vi "nanocal -- nuclear schottky goodness V6.vi"(5 "action":T1=enum."onlygrads", 6 "parameters IN":map{T2, dbl}(c390), 7 "weighting strategy":T3, 8 "dz/dω IN (V)":cdb[](array[numeric])=[1.7183506006211996e-05+0.0i, 1.7124360968751133e-05+0.0i, 1.7049104347380084e-05+0.0i, 1.700437896335042e-05+0.0i, 1.6984579723285106e-05+0.0i, 1.702277369054923e-05+0.0i, 1.713094025845651e-05+0.0i, 1.734249707866828e-05+0.0i, 1.768320429215342e-05+0.0i, 1.8195281152538477e-05+0.0i, 1.8917228661806973e-05+0.0i, 1.9897834564883332e-05+0.0i, 2.154104046962704e-05+0.0i, 2.3247799321765792e-05+0.0i, 2.5364678450551808e-05+0.0i, 2.8645788781885885e-05+0.0i, 3.204749554800641e-05+0.0i, 3.783559691555022e-05+0.0i, 4.245015867332296e-05+0.0i, 4.909131821431355e-05+0.0i, 5.511821898441184e-05+0.0i, 6.178843506022867e-05+0.0i, 7.1079604965352e-05+0.0i, 7.922304381453334e-05+0.0i, 8.814778883893872e-05+0.0i, 9.806709148886077e-05+0.0i, 0.00011119043245647465+0.0i, 0.00012253184919712196+0.0i, 0.00013777724317049346+0.0i, 0.0001508081004573332+0.0i, 0.00016547294918783876+0.0i, 0.00018003847596605868+0.0i, 0.00019518361086534857+0.0i, 0.00021134179818259658+0.0i, 0.0002372041782935464+0.0i, 0.00025518143132024254+0.0i, 0.0002835129702467886+0.0i, 0.0003060118087631287+0.0i, 0.00032860772064336976+0.0i, 0.0003492674091322389+0.0i, 0.00037498324855458583+0.0i, 0.00040021078021115026+0.0i, 0.00041969942568205823+0.0i, 0.00044367338947118773+0.0i, 0.0004634793607238068+0.0i, 0.00047921028781215815+0.0i, 0.0004880906353641744+0.0i, 0.0004932212623741357+0.0i, 0.000491476456593048+0.0i, 0.000480893803992059+0.0i, 0.0004535995818650303+0.0i, 0.000417087772881063+0.0i, 0.0003564148692854789+0.0i, 0.0003049201646356487+0.0i, 0.00021260191240459413+0.0i, 0.00011714858948470126+0.0i, 1.675457544365132e-05+0.0i, -6.8674075405897e-05+0.0i, -0.000156473047607305+0.0i, -0.00026709373934749337+0.0i, -0.0003544271565676041+0.0i, -0.00047937600197311275+0.0i, -0.0006086290582260493+0.0i, -0.0007031877411848573+0.0i, -0.0007564526901441745+0.0i, -0.000802489180995596+0.0i, -0.0008414596018105983+0.0i, -0.0008809346482248761+0.0i, -0.0009073902840241921+0.0i, -0.0009264953054508651+0.0i, -0.0009405659412141811+0.0i, -0.000951649722530156+0.0i, -0.0009557485581057351+0.0i, -0.0009558464741053665+0.0i, -0.0009509110176922098+0.0i, -0.0009411315169847015+0.0i, -0.0009303400913929496+0.0i, -0.0009171113529290538+0.0i, -0.0009022111527275027+0.0i, -0.0008813746494947608+0.0i, -0.0008581837971946129+0.0i, -0.0008372063466683705+0.0i, -0.0008165626610594428+0.0i, -0.0007901155435838691+0.0i, -0.0007682834352800848+0.0i, -0.000746231015527196+0.0i, -0.0007238798463130141+0.0i, -0.0007015567569177018+0.0i, -0.000679301954671598+0.0i, -0.0006572001413831251+0.0i, -0.000629855254567978+0.0i, -0.0006083942229188815+0.0i, -0.0005768631156754208+0.0i, -0.0005562177438951648+0.0i, -0.0005359092039599222+0.0i, -0.0005145186443378148+0.0i, -0.0004951602053444319+0.0i, -0.00047624970229075174+0.0i, -0.0004577401041527736+0.0i, -0.00043519037796120065+0.0i], 9 "Voltage IN (V)":cdb[](array[numeric])=[1.7183506006211996e-05+0.0i, 1.7124360968751133e-05+0.0i, 1.7049104347380084e-05+0.0i, 1.700437896335042e-05+0.0i, 1.6984579723285106e-05+0.0i, 1.702277369054923e-05+0.0i, 1.713094025845651e-05+0.0i, 1.734249707866828e-05+0.0i, 1.768320429215342e-05+0.0i, 1.8195281152538477e-05+0.0i, 1.8917228661806973e-05+0.0i, 1.9897834564883332e-05+0.0i, 2.154104046962704e-05+0.0i, 2.3247799321765792e-05+0.0i, 2.5364678450551808e-05+0.0i, 2.8645788781885885e-05+0.0i, 3.204749554800641e-05+0.0i, 3.783559691555022e-05+0.0i, 4.245015867332296e-05+0.0i, 4.909131821431355e-05+0.0i, 5.511821898441184e-05+0.0i, 6.178843506022867e-05+0.0i, 7.1079604965352e-05+0.0i, 7.922304381453334e-05+0.0i, 8.814778883893872e-05+0.0i, 9.806709148886077e-05+0.0i, 0.00011119043245647465+0.0i, 0.00012253184919712196+0.0i, 0.00013777724317049346+0.0i, 0.0001508081004573332+0.0i, 0.00016547294918783876+0.0i, 0.00018003847596605868+0.0i, 0.00019518361086534857+0.0i, 0.00021134179818259658+0.0i, 0.0002372041782935464+0.0i, 0.00025518143132024254+0.0i, 0.0002835129702467886+0.0i, 0.0003060118087631287+0.0i, 0.00032860772064336976+0.0i, 0.0003492674091322389+0.0i, 0.00037498324855458583+0.0i, 0.00040021078021115026+0.0i, 0.00041969942568205823+0.0i, 0.00044367338947118773+0.0i, 0.0004634793607238068+0.0i, 0.00047921028781215815+0.0i, 0.0004880906353641744+0.0i, 0.0004932212623741357+0.0i, 0.000491476456593048+0.0i, 0.000480893803992059+0.0i, 0.0004535995818650303+0.0i, 0.000417087772881063+0.0i, 0.0003564148692854789+0.0i, 0.0003049201646356487+0.0i, 0.00021260191240459413+0.0i, 0.00011714858948470126+0.0i, 1.675457544365132e-05+0.0i, -6.8674075405897e-05+0.0i, -0.000156473047607305+0.0i, -0.00026709373934749337+0.0i, -0.0003544271565676041+0.0i, -0.00047937600197311275+0.0i, -0.0006086290582260493+0.0i, -0.0007031877411848573+0.0i, -0.0007564526901441745+0.0i, -0.000802489180995596+0.0i, -0.0008414596018105983+0.0i, -0.0008809346482248761+0.0i, -0.0009073902840241921+0.0i, -0.0009264953054508651+0.0i, -0.0009405659412141811+0.0i, -0.000951649722530156+0.0i, -0.0009557485581057351+0.0i, -0.0009558464741053665+0.0i, -0.0009509110176922098+0.0i, -0.0009411315169847015+0.0i, -0.0009303400913929496+0.0i, -0.0009171113529290538+0.0i, -0.0009022111527275027+0.0i, -0.0008813746494947608+0.0i, -0.0008581837971946129+0.0i, -0.0008372063466683705+0.0i, -0.0008165626610594428+0.0i, -0.0007901155435838691+0.0i, -0.0007682834352800848+0.0i, -0.000746231015527196+0.0i, -0.0007238798463130141+0.0i, -0.0007015567569177018+0.0i, -0.000679301954671598+0.0i, -0.0006572001413831251+0.0i, -0.000629855254567978+0.0i, -0.0006083942229188815+0.0i, -0.0005768631156754208+0.0i, -0.0005562177438951648+0.0i, -0.0005359092039599222+0.0i, -0.0005145186443378148+0.0i, -0.0004951602053444319+0.0i, -0.00047624970229075174+0.0i, -0.0004577401041527736+0.0i, -0.00043519037796120065+0.0i], 10 "ω (rad/sec)":dbl[](array[numeric])=[32012.991918577427, 32390.261658505893, 32466.39798177853, 32499.14340521798, 32517.39286113775, 32529.046092051318, 32537.14525712326, 32543.111142615544, 32547.696343954158, 32551.33675949651, 32554.302325209504, 32556.769142360055, 32558.856995237307, 32560.650202739795, 32562.209843476354, 32563.58125099723, 32564.7987833122, 32565.88895894197, 32566.872575330308, 32567.766175404246, 32568.583086316496, 32569.334166794306, 32570.02835688638, 32570.673085530187, 32571.274580490695, 32571.838104118455, 32572.36813539066, 32572.868514009202, 32573.342552524307, 32573.793126289274, 32574.222746575288, 32574.633618125405, 32575.027687968828, 32575.40668442971, 32575.772149741057, 32576.12546690325, 32576.467883345118, 32576.800529469096, 32577.124435064776, 32577.440543590797, 32577.749724325146, 32578.052781957467, 32578.35046682089, 32578.643482565894, 32578.932492128843, 32579.218126471686, 32579.500987779396, 32579.781656707495, 32580.06069600583, 32580.338656060805, 32580.616078519142, 32580.89350097748, 32581.171461032456, 32581.45050033079, 32581.73116925889, 32582.0140305666, 32582.29966469628, 32582.58867447239, 32582.88169000423, 32583.179375080817, 32583.48243271314, 32583.791613234323, 32584.10772197351, 32584.43162756919, 32584.764273480003, 32585.106690135035, 32585.460007297228, 32585.825472395412, 32586.204468856296, 32586.59853891288, 32587.009410462997, 32587.439030535847, 32587.889604513977, 32588.363642815923, 32588.86402143446, 32589.39405291983, 32589.957576334426, 32590.559071508098, 32591.203800151903, 32591.897990030815, 32592.64907072179, 32593.46598163404, 32594.359581707977, 32595.343197883154, 32596.433373726086, 32597.650906041054, 32599.022313348767, 32600.58195429849, 32602.375161800977, 32604.46301467823, 32606.929831615616, 32609.895397541775, 32613.535812870963, 32618.12101442274, 32624.086899701866, 32632.186064986967, 32643.839295900536, 32662.088751820305, 32694.834175046595, 32770.97049853239]) -> (0 "R norm":dbl=-1.0, 1 "G":dbl=-1.0, 2 "R(ω) out":cdb[](array[numeric])=[1.7183506006211996e-05+0.0i, 1.7124360968751133e-05+0.0i, 1.7049104347380084e-05+0.0i, 1.700437896335042e-05+0.0i, 1.6984579723285106e-05+0.0i, 1.702277369054923e-05+0.0i, 1.713094025845651e-05+0.0i, 1.734249707866828e-05+0.0i, 1.768320429215342e-05+0.0i, 1.8195281152538477e-05+0.0i, 1.8917228661806973e-05+0.0i, 1.9897834564883332e-05+0.0i, 2.154104046962704e-05+0.0i, 2.3247799321765792e-05+0.0i, 2.5364678450551808e-05+0.0i, 2.8645788781885885e-05+0.0i, 3.204749554800641e-05+0.0i, 3.783559691555022e-05+0.0i, 4.245015867332296e-05+0.0i, 4.909131821431355e-05+0.0i, 5.511821898441184e-05+0.0i, 6.178843506022867e-05+0.0i, 7.1079604965352e-05+0.0i, 7.922304381453334e-05+0.0i, 8.814778883893872e-05+0.0i, 9.806709148886077e-05+0.0i, 0.00011119043245647465+0.0i, 0.00012253184919712196+0.0i, 0.00013777724317049346+0.0i, 0.0001508081004573332+0.0i, 0.00016547294918783876+0.0i, 0.00018003847596605868+0.0i, 0.00019518361086534857+0.0i, 0.00021134179818259658+0.0i, 0.0002372041782935464+0.0i, 0.00025518143132024254+0.0i, 0.0002835129702467886+0.0i, 0.0003060118087631287+0.0i, 0.00032860772064336976+0.0i, 0.0003492674091322389+0.0i, 0.00037498324855458583+0.0i, 0.00040021078021115026+0.0i, 0.00041969942568205823+0.0i, 0.00044367338947118773+0.0i, 0.0004634793607238068+0.0i, 0.00047921028781215815+0.0i, 0.0004880906353641744+0.0i, 0.0004932212623741357+0.0i, 0.000491476456593048+0.0i, 0.000480893803992059+0.0i, 0.0004535995818650303+0.0i, 0.000417087772881063+0.0i, 0.0003564148692854789+0.0i, 0.0003049201646356487+0.0i, 0.00021260191240459413+0.0i, 0.00011714858948470126+0.0i, 1.675457544365132e-05+0.0i, -6.8674075405897e-05+0.0i, -0.000156473047607305+0.0i, -0.00026709373934749337+0.0i, -0.0003544271565676041+0.0i, -0.00047937600197311275+0.0i, -0.0006086290582260493+0.0i, -0.0007031877411848573+0.0i, -0.0007564526901441745+0.0i, -0.000802489180995596+0.0i, -0.0008414596018105983+0.0i, -0.0008809346482248761+0.0i, -0.0009073902840241921+0.0i, -0.0009264953054508651+0.0i, -0.0009405659412141811+0.0i, -0.000951649722530156+0.0i, -0.0009557485581057351+0.0i, -0.0009558464741053665+0.0i, -0.0009509110176922098+0.0i, -0.0009411315169847015+0.0i, -0.0009303400913929496+0.0i, -0.0009171113529290538+0.0i, -0.0009022111527275027+0.0i, -0.0008813746494947608+0.0i, -0.0008581837971946129+0.0i, -0.0008372063466683705+0.0i, -0.0008165626610594428+0.0i, -0.0007901155435838691+0.0i, -0.0007682834352800848+0.0i, -0.000746231015527196+0.0i, -0.0007238798463130141+0.0i, -0.0007015567569177018+0.0i, -0.000679301954671598+0.0i, -0.0006572001413831251+0.0i, -0.000629855254567978+0.0i, -0.0006083942229188815+0.0i, -0.0005768631156754208+0.0i, -0.0005562177438951648+0.0i, -0.0005359092039599222+0.0i, -0.0005145186443378148+0.0i, -0.0004951602053444319+0.0i, -0.00047624970229075174+0.0i, -0.0004577401041527736+0.0i, -0.00043519037796120065+0.0i], 3 "dG / d log α   OUT":map{T2, dbl}(c390), 4 "d2G / d log α d log  β  map  OUT":map{i32[], dbl}(c390))   [LabVIEW 2021]
uses:
  nanocal-goodness-weighting-strategy.ctl
  3-lorentzian-parameters.ctl
  3-lorentzian-heat-response action.ctl
  <vilib>/Utility/miscctls.llb/LVMapReplaceAction.ctl
  <vilib>/Analysis/_algsub.llb/Matrix Norm Type.ctl
  <vilib>/Analysis/baseanly.llb/Matrix Type of Inverse Matrix.ctl
  <vilib>/Analysis/baseanly.llb/Real A x B.vi
  <vilib>/Analysis/_algsub.llb/Real Matrix Norm.vi
  <vilib>/Analysis/Matrix/Numeric/Conversions/Array To Matrix - RA2.vi
  <vilib>/Analysis/baseanly.llb/Real Inverse Matrix.vi
  <vilib>/Analysis/Matrix/Numeric/Conversions/Array To Matrix - RA.vi
  <vilib>/Analysis/Matrix/Numeric/Conversions/Matrix To Array - RM.vi
  <vilib>/Analysis/Matrix/NI_Matrix.lvlib
  <vilib>/Analysis/NI_AALBase.lvlib
  <vilib>/Analysis/NI_AALPro.lvlib
panel:
  out "d2G / d log α d log  β  matrix OUT":dbl[](array[numeric])
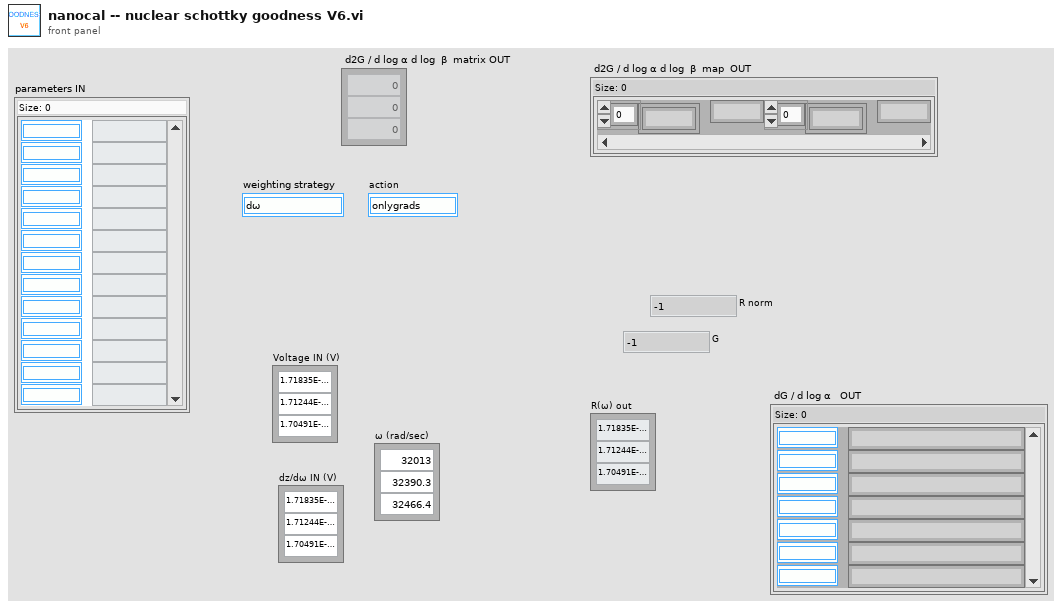
[diagram p1: front panel]
types:
  T1 = typedef "3-lorentzian-heat-response action.ctl" = enum16{"calc R", "create string", "calc m1m2m3", "dζ", "dT1", "dτS", "dτN", "dτC", "d-all", "dκ0", "T(K)", "m1", "m2", "m3", "parse string", "θ (deg)", "B (T)", "onlygrads", "newton", "create emty string", "simple2nd", "calc R2"}
  T2 = typedef "3-lorentzian-parameters.ctl" = enum16{"ζ", "τ1", "τS", "τN", "τC", "κ0", "m1", "m2", "m3", "T (K)", "B (T)", "θ (deg)", "side (S|R)", "set of (B|T)", "Re(offset)", "Im(offset)", "στ1", "στ1-", "στ1+", "στS", "στS-", "στS+", "στN", "στN-", "στN+", "τ11", "τ12", "τ21", "τ22", "τN1", "τN2"}
  T3 = typedef "nanocal-goodness-weighting-strategy.ctl" = enum16{"dω", "dω √(|dz/dω|)", "dω |dz/dω|", "phase", "andreas", "sum", "anti-andr", "ark"}
  T4 = typedef "LVMapReplaceAction.ctl" = enum32{"Modify Entry only if found", "Add or Modify Entry", "Delete Entry"}
  T5 = typedef "NI_AALBase.lvlib/Matrix Type of Inverse Matrix.ctl" = enum32{"General", "Positive Definite", "Lower Triangular", "Upper Triangular"}
  T6 = typedef "NI_AALPro.lvlib/Matrix Norm Type.ctl" = i32
  T7 = typedef "NI_Matrix.lvlib/RealMatrix.ctl" = dbl[][]
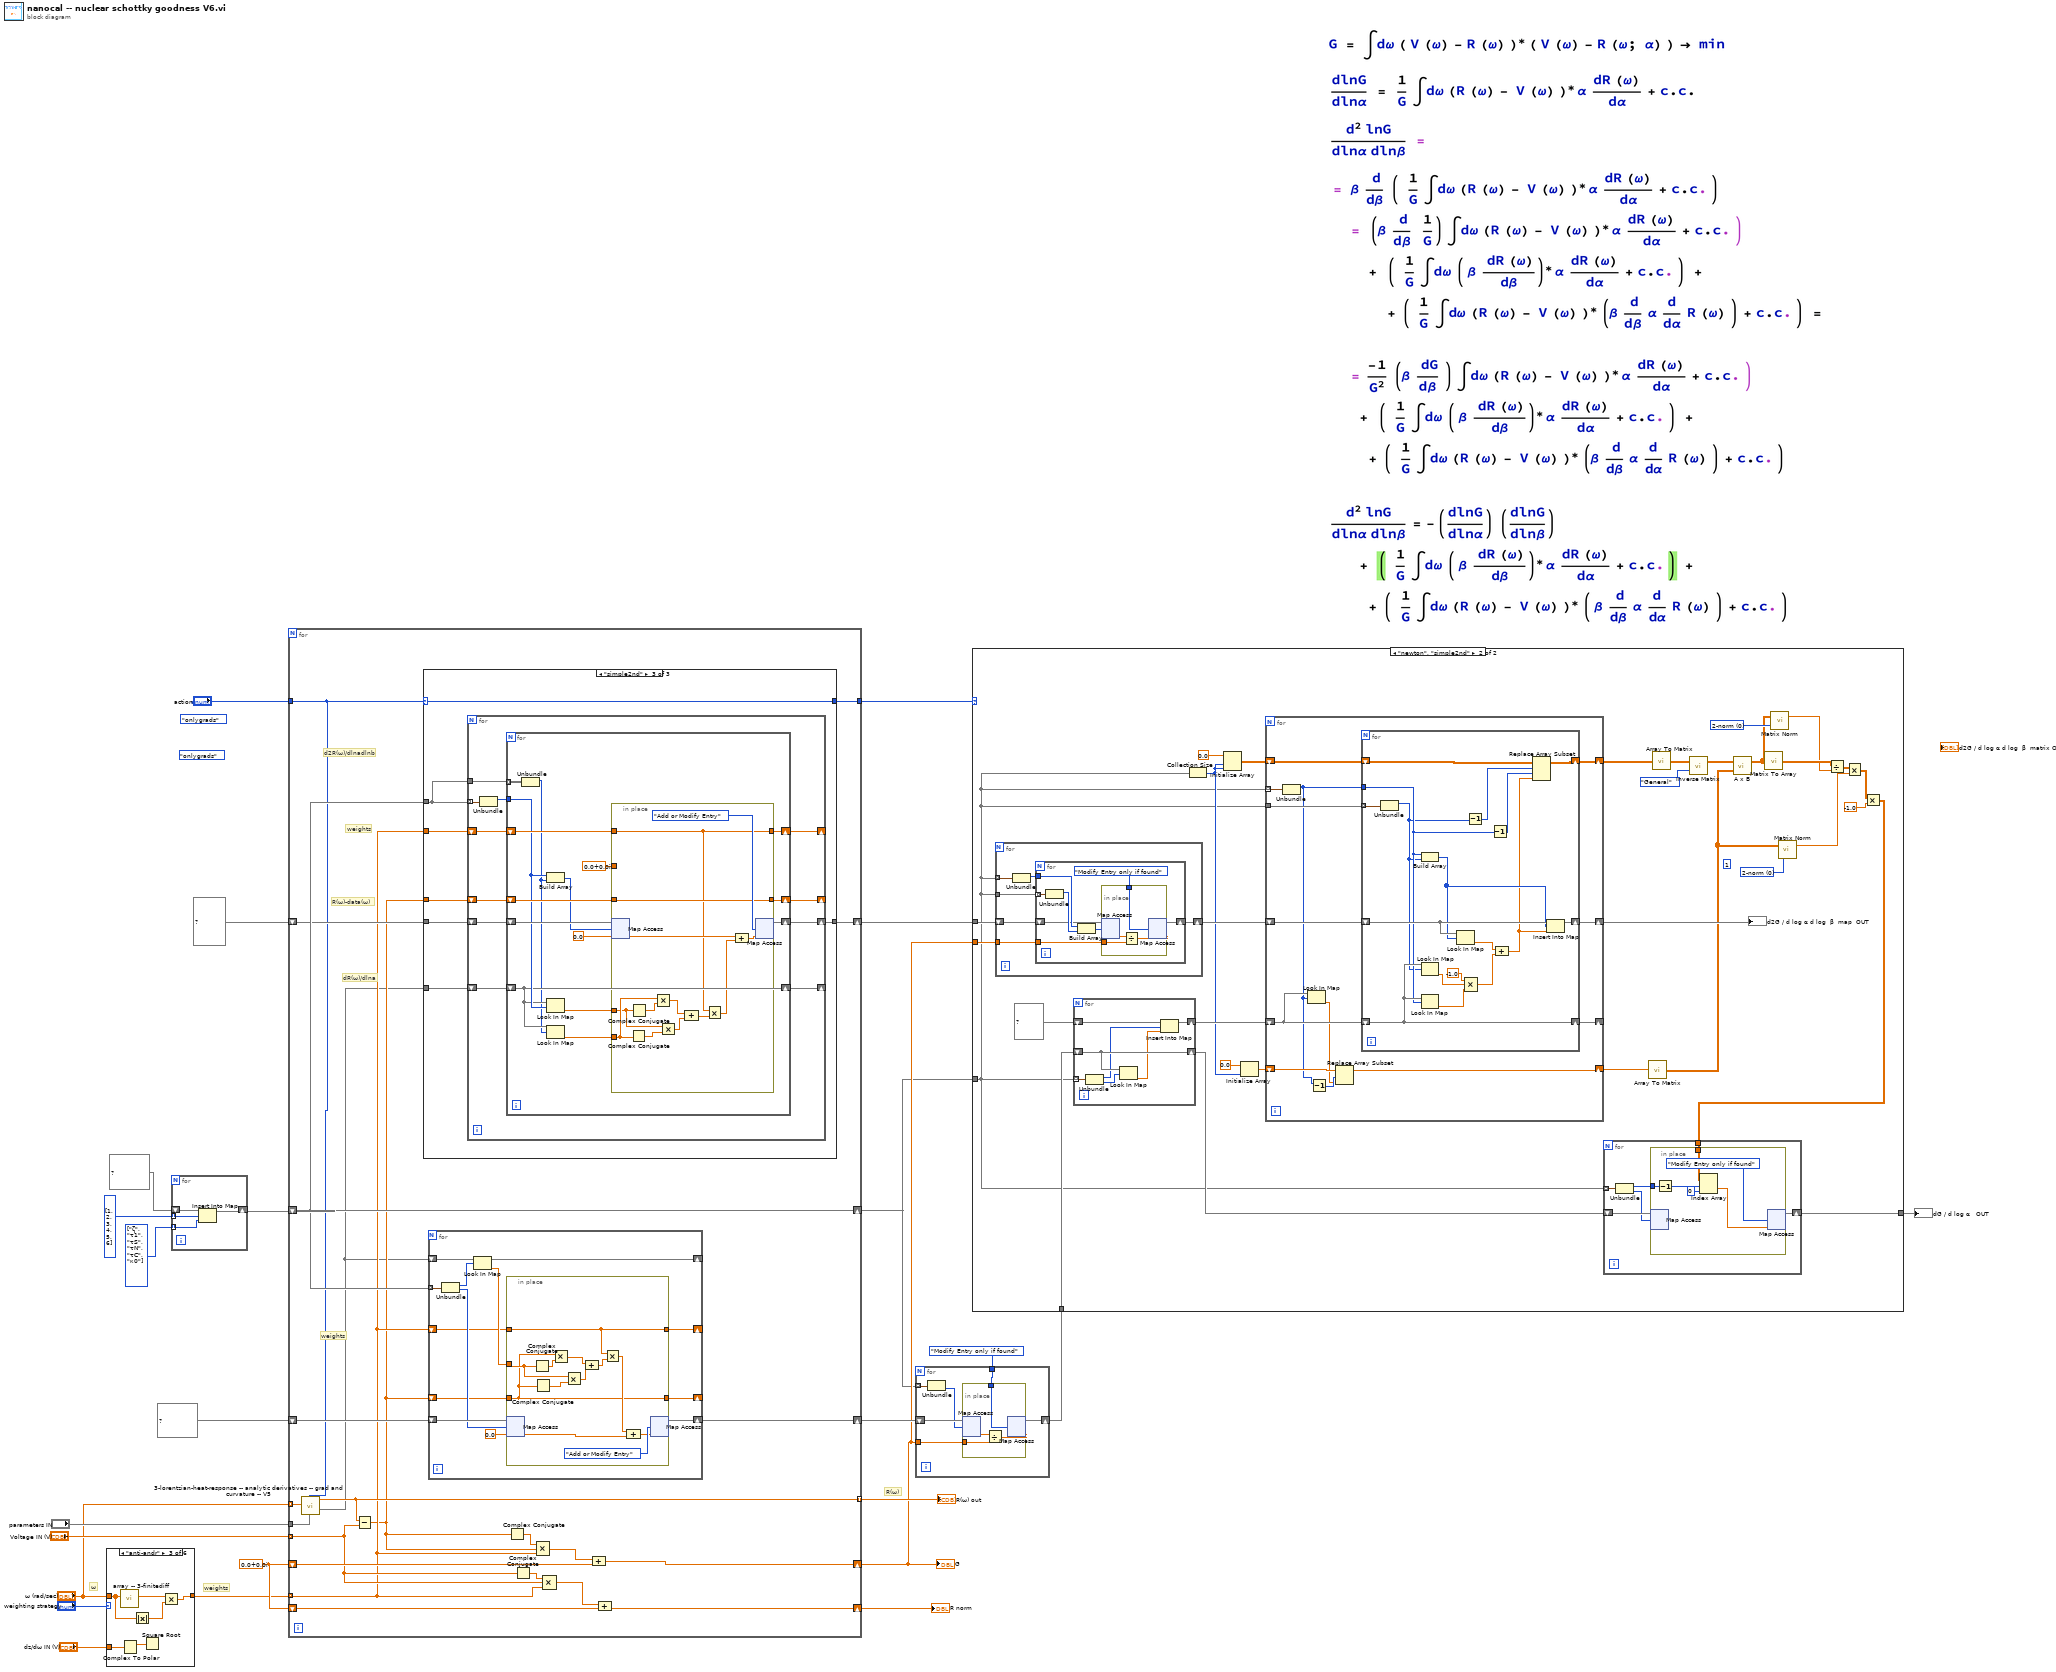
[diagram p0: block diagram]
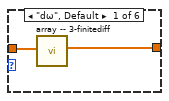
[diagram p3: hidden frame]
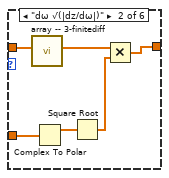
[diagram p4: hidden frame]
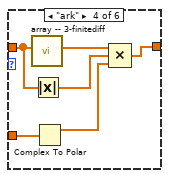
[diagram p5: hidden frame]
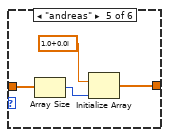
[diagram p6: hidden frame]
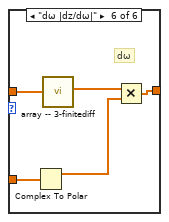
[diagram p7: hidden frame]
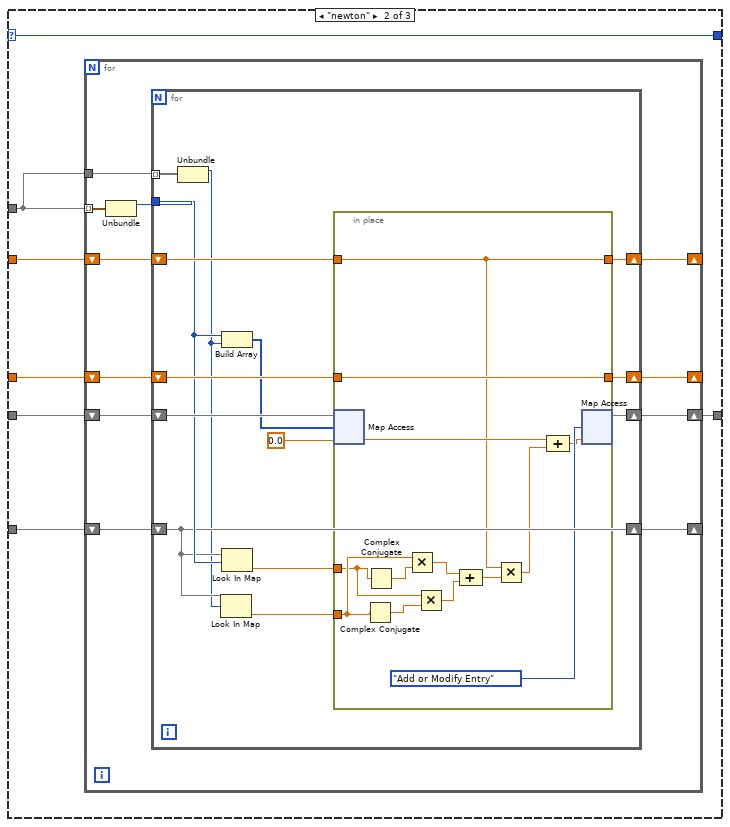
[diagram p9: hidden frame]
diagram:
  (unwired) 3-lorentzian-heat-response_action."onlygrads" ("action")
  (unwired) 3-lorentzian-heat-response_action."onlygrads" ("action")
  w14 = cdb 0.0+0.0i ("y")
  w19 = T2[] [enum."ζ", enum."τ1", enum."τS", enum."τN", enum."τC", enum."κ0"] items=["ζ", "τ1", "τS", "τN", "τC", "κ0", "m1", "m2", "m3", "T (K)", "B (T)", "θ (deg)", "side (S|R)", "set of (B|T)", "Re(offset)", "Im(offset)", "στ1", "στ1-", "στ1+", "στS", "στS-", "στS+", "στN", "στN-", "στN+", "τ11", "τ12", "τ21", "τ22", "τN1", "τN2"]
  # "weights"
  # "R(ω)"
  # "ω"
  n1 = case shown="\"anti-andr\"" "weighting strategy" {
    tunnel: "dz/dω IN (V)" -> [_ w32 w38 w44 _ w53]
    tunnel: "ω (rad/sec)" -> [w26 w28 w34 w41 w48 w52]
    tunnel: [w25 w27 w35 w42 w45 w49] -> w3
    frame "dω", Default {
      n2 = call "array -- 3-finitediff.vi"("ω (rad/sec)"=w26) -> ("dω (rad/sec)"=w25:cdb[])  [unwired: 10 in]
    }
    frame "dω √(|dz/dω|)" {
      n3 = call "array -- 3-finitediff.vi"("ω (rad/sec)"=w28) -> ("dω (rad/sec)"=w30:cdb[])  [unwired: 10 in]
      n4 = Complex To Polar(r * e^(i*theta)=w32) -> (r=w31:dbl[])  [unwired: 1 out]
      n5 = Square Root(x=w31) -> (sqrt(x)=w29:dbl[])
      n6 = Multiply(x=w30, y=w29) -> (x*y=w27:cdb[])
    }
    frame "anti-andr" {
      n7 = call "array -- 3-finitediff.vi"("ω (rad/sec)"=w34) -> ("dω (rad/sec)"=w36:cdb[])  [unwired: 10 in]
      n8 = Complex To Polar(r * e^(i*theta)=w38) -> (r=w37:dbl[])  [unwired: 1 out]
      n9 = Absolute Value(x=w34) -> (abs(x)=w33:dbl[])
      n10 = Square Root(x=w37) -> ()  [unwired: 1 out]
      n11 = Multiply(x=w36, y=w33) -> (x*y=w35:cdb[])
    }
    frame "ark" {
      n12 = call "array -- 3-finitediff.vi"("ω (rad/sec)"=w41) -> ("dω (rad/sec)"=w43:cdb[])  [unwired: 10 in]
      n13 = Absolute Value(x=w41) -> (abs(x)=w40:dbl[])
      n14 = Complex To Polar(r * e^(i*theta)=w44) -> (r=w39:dbl[])  [unwired: 1 out]
      n15 = Compound Arithmetic op=MULTIPLY(w43, w40, w39) -> (w42:cdb[])
    }
    frame "andreas" {
      n16 = Array Size(array=w48) -> (size(s)=w47:i32)
      n17 = Initialize Array(cdb 1.0+0.0i ("y"), w47) -> (w45:cdb[])
    }
    frame "dω |dz/dω|" {
      # "dω"
      n18 = Complex To Polar(r * e^(i*theta)=w53) -> (r=w51:dbl[])  [unwired: 1 out]
      n19 = call "array -- 3-finitediff.vi"("ω (rad/sec)"=w52) -> ("dω (rad/sec)"=w50:cdb[])  [unwired: 10 in]
      n20 = Multiply(x=w50, y=w51) -> (x*y=w49:cdb[])
    }
  }
  n21 = for {
    tunnel: w19 -> [w54] mode=indexing
    shift-right: [w56] -> w12
    shift-left: map{i32, T2} {} ("parameters IN") -> [w57]
    tunnel: i32[] [1, 2, 3, 4, 5, 6] -> [w55] mode=indexing
    n22 = Insert Into Map(map in=w57, key=w55, value=w54) -> (map out=w56:map{i32, T2})  [unwired: 2 out]
  }
  n23 = for {
    tunnel: "ω (rad/sec)" -> [w78] mode=indexing
    tunnel: [w77] -> w21 mode=indexing
    tunnel: "parameters IN" -> [w79]
    tunnel: "Voltage IN (V)" -> [w66] mode=indexing
    tunnel: w3 -> [w62] mode=indexing
    shift-right: [w75] -> w15
    shift-left: map{T2, dbl} {} ("parameters IN") -> [w76]
    shift-right: [w65] -> w7
    shift-left: w12 -> [w65]
    shift-right: [w71] -> w8
    shift-left: w14 -> [w72]
    shift-right: [w67] -> w13
    shift-left: w14 -> [w68]
    shift-right: [w63] -> w9
    shift-left: map{i32[], dbl} {} ("parameters IN") -> [w64]
    tunnel: "action" -> [w59]
    tunnel: [w58] -> w5
    # "R(ω)-data(ω)"
    # "weights"
    # "dR(ω)/dlna"
    # "d2R(ω)/dlnadlnb"
    # "weights"
    n24 = call "3-lorentzian-heat-response -- analytic derivatives -- grad and curvature -- V5.vi"("parameters map  IN"=w79, "action"=w59, "ω (rad/sec)"=w78) -> ("grad map  out"=w60:map{i32, cdb}, "R(ω)"=w77:cdb)  [unwired: 6 in, 1 out]
    n25 = Subtract(x=w77, y=w66) -> (x-y=w61:cdb)
    n26 = case shown="\"simple2nd\"" w59 {
      selector: w59 -> [w80 w82 w127]
      tunnel: w65 -> [_ w88 w133]
      tunnel: w64 -> [w81 w87 w132]
      tunnel: [w81 w86 w131] -> w63
      tunnel: w62 -> [_ w85 w130]
      tunnel: w61 -> [_ w84 w129]
      tunnel: w60 -> [_ w83 w128]
      tunnel: [w80 w82 w127] -> w58
      frame "calc R", Default {
      }
      frame "newton" {
        n27 = for {
          shift-right: [w99] -> w86
          shift-left: w87 -> [w98]
          shift-right: [w97] -> _
          shift-left: w85 -> [w95]
          shift-right: [w96] -> _
          shift-left: w84 -> [w94]
          tunnel: w88 -> [w93] mode=indexing
          tunnel: w88 -> [w92]
          shift-right: [w89] -> _
          shift-left: w83 -> [w90]
          n28 = Unbundle(w93) -> ("index"=w91:i32)  [unwired: 1 out]
          n29 = for {
            shift-right: [w111] -> w96
            shift-left: w94 -> [w110]
            shift-right: [w109] -> w99
            shift-left: w98 -> [w113]
            tunnel: w92 -> [w106] mode=indexing
            shift-right: [w107] -> w97
            shift-left: w95 -> [w108]
            tunnel: w91 -> [w104]
            shift-right: [w103] -> w89
            shift-left: w90 -> [w103]
            n30 = Unbundle(w106) -> ("index"=w102:i32)  [unwired: 1 out]
            n31 = Look In Map(map=w103, key=w102) -> (value=w100:cdb)  [unwired: 1 in, 1 out]
            n32 = Build Array(w104, w102) -> (w105:i32[])
            n33 = Look In Map(map=w103, key=w104) -> (value=w101:cdb)  [unwired: 1 in, 1 out]
            n34 = in-place {
              in-place-border: [w123] -> w111
              in-place-border: w110 -> [w123]
              in-place-border: w108 -> [w114]
              in-place-border: [w114] -> w107
              in-place-border: w101 -> [w116]
              in-place-border: w100 -> [w117]
              n35 = in-place-map #1(w113, w105, 0.0 ("number")) -> (w125:dbl)  [unwired: 1 out]
              n36 = Complex Conjugate(1:w117) -> (0:w121:cdb)
              n37 = Complex Conjugate(1:w116) -> (0:w122:cdb)
              n38 = Multiply(x=w117, y=w122) -> (x*y=w120:cdb)
              n39 = Multiply(x=w116, y=w121) -> (x*y=w119:cdb)
              n40 = Compound Arithmetic op=ADD(w120, w119) -> (w118:cdb)
              n41 = Multiply(x=w114, y=w118) -> (x*y=w115:cdb)
              n42 = Compound Arithmetic op=ADD(w125, w115) -> (w124:cdb)
              n43 = in-place-map #1(w124, LVMapReplaceAction."Add or Modify Entry" ("action")) -> (w109:map{i32[], dbl})  [unwired: 2 out]
            }
          }
        }
      }
      frame "simple2nd" {
        n44 = for {
          shift-right: [w144] -> w131
          shift-left: w132 -> [w143]
          shift-right: [w142] -> _
          shift-left: w130 -> [w140]
          shift-right: [w141] -> _
          shift-left: w129 -> [w139]
          tunnel: w133 -> [w138] mode=indexing
          tunnel: w133 -> [w137]
          shift-right: [w134] -> _
          shift-left: w128 -> [w135]
          n45 = Unbundle(w138) -> ("index"=w136:i32)  [unwired: 1 out]
          n46 = for {
            shift-right: [w157] -> w141
            shift-left: w139 -> [w156]
            shift-right: [w155] -> w144
            shift-left: w143 -> [w159]
            tunnel: w137 -> [w152] mode=indexing
            shift-right: [w153] -> w142
            shift-left: w140 -> [w154]
            tunnel: w136 -> [w150]
            shift-right: [w149] -> w134
            shift-left: w135 -> [w149]
            n47 = Unbundle(w152) -> ("index"=w148:i32)  [unwired: 1 out]
            n48 = Look In Map(map=w149, key=w148) -> (value=w146:cdb)  [unwired: 1 in, 1 out]
            n49 = Build Array(w150, w148) -> (w151:i32[])
            n50 = Look In Map(map=w149, key=w150) -> (value=w147:cdb)  [unwired: 1 in, 1 out]
            n51 = in-place {
              in-place-border: [w169] -> w157
              in-place-border: w156 -> [w169]
              in-place-border: cdb 0.0+0.0i -> [_]
              in-place-border: w154 -> [w161]
              in-place-border: [w161] -> w153
              in-place-border: w147 -> [w162]
              in-place-border: w146 -> [w163]
              n52 = in-place-map #2(w159, w151, 0.0 ("number")) -> (w171:dbl)  [unwired: 1 out]
              n53 = Complex Conjugate(1:w163) -> (0:w167:cdb)
              n54 = Complex Conjugate(1:w162) -> (0:w168:cdb)
              n55 = Multiply(x=w163, y=w168) -> (x*y=w166:cdb)
              n56 = Multiply(x=w162, y=w167) -> (x*y=w165:cdb)
              n57 = Compound Arithmetic op=ADD(w166, w165) -> (w164:cdb)
              n58 = Multiply(x=w161, y=w164) -> (x*y=w160:cdb)
              n59 = Compound Arithmetic op=ADD(w171, w160) -> (w170:cdb)
              n60 = in-place-map #2(w170, LVMapReplaceAction."Add or Modify Entry" ("action")) -> (w155:map{i32[], dbl})  [unwired: 2 out]
            }
          }
        }
      }
    }
    n61 = for {
      shift-right: [w184] -> _
      shift-left: w60 -> [w184]
      shift-right: [w178] -> _
      shift-left: w61 -> [w177]
      shift-right: [w175] -> w75
      shift-left: w76 -> [w181]
      tunnel: w65 -> [w183] mode=indexing
      shift-right: [w173] -> _
      shift-left: w62 -> [w174]
      n62 = Unbundle(w183) -> ("index"=w182:i32, "X selector"=w180:T2)
      n63 = Look In Map(map=w184, key=w182) -> (value=w176:cdb)  [unwired: 1 in, 1 out]
      n64 = in-place {
        in-place-border: [w186] -> w178
        in-place-border: w177 -> [w186]
        in-place-border: w176 -> [w193]
        in-place-border: w174 -> [w185]
        in-place-border: [w185] -> w173
        n65 = in-place-map #3(w181, w180, 0.0 ("number")) -> (w192:dbl)  [unwired: 1 out]
        n66 = Complex Conjugate(1:w193) -> (0:w195:cdb)
        n67 = Complex Conjugate(1:w186) -> (0:w194:cdb)
        n68 = Multiply(x=w186, y=w195) -> (x*y=w190:cdb)
        n69 = Multiply(x=w193, y=w194) -> (x*y=w189:cdb)
        n70 = Compound Arithmetic op=ADD(w190, w189) -> (w188:cdb)
        n71 = Multiply(x=w185, y=w188) -> (x*y=w187:cdb)
        n72 = Compound Arithmetic op=ADD(w187, w192) -> (w191:cdb)
        n73 = in-place-map #3(w191, LVMapReplaceAction."Add or Modify Entry" ("action")) -> (w175:map{T2, dbl})  [unwired: 2 out]
      }
    }
    n74 = Complex Conjugate(1:w61) -> (0:w74:cdb)
    n75 = Complex Conjugate(1:w66) -> (0:w70:cdb)
    n76 = Compound Arithmetic op=MULTIPLY(w74, w61, w62) -> (w73:cdb)
    n77 = Compound Arithmetic op=MULTIPLY(w70, w66, w62) -> (w69:cdb)
    n78 = Compound Arithmetic op=ADD(w73, w72) -> (w71:cdb)
    n79 = Compound Arithmetic op=ADD(w69, w68) -> (w67:cdb)
  }
  "G" <- w8
  "R norm" <- w13
  "R(ω) out" <- w21
  n80 = for {
    tunnel: w7 -> [w199] mode=indexing
    shift-right: [w201] -> w10
    shift-left: w15 -> [w202]
    tunnel: w8 -> [w200]
    tunnel: LVMapReplaceAction."Modify Entry only if found" ("action") -> [w197]
    n81 = Unbundle(w199) -> ("X selector"=w198:T2)  [unwired: 1 out]
    n82 = in-place {
      in-place-border: w200 -> [w205]
      in-place-border: w197 -> [w203]
      n83 = in-place-map #4(w202, w198) -> (w206:dbl)  [unwired: 1 in, 1 out]
      n84 = Divide(x=w206, y=w205) -> (x/y=w204:cdb)
      n85 = in-place-map #4(w204, w203) -> (w201:map{T2, dbl})  [unwired: 2 out]
    }
  }
  n86 = case shown="\"newton\", \"simple2nd\"" w5 {
    tunnel: w10 -> [w207 w237]
    tunnel: w9 -> [_ w236]
    tunnel: w8 -> [_ w234]
    tunnel: w7 -> [_ w216]
    tunnel: [w207 w215] -> w6
    frame "calc R", Default {
    }
    frame "newton", "simple2nd" {
      w222 = T6 0 items=["2-norm", "1-norm", "F-norm", "Inf-norm"] ("norm type")
      w223 = T6 0 items=["2-norm", "1-norm", "F-norm", "Inf-norm"] ("norm type")
      (unwired) 1 ("number of columns")
      n87 = for {
        tunnel: w216 -> [w255] mode=indexing
        tunnel: w216 -> [w256]
        shift-right: [w252] -> w235
        shift-left: w236 -> [w253]
        tunnel: w234 -> [w251]
        n88 = Unbundle(w255) -> ("index"=w254:i32)  [unwired: 1 out]
        n89 = for {
          tunnel: w256 -> [w264] mode=indexing
          tunnel: w254 -> [w263]
          shift-right: [w260] -> w252
          shift-left: w253 -> [w261]
          tunnel: w251 -> [w258]
          n90 = Unbundle(w264) -> ("index"=w262:i32)  [unwired: 1 out]
          n91 = Build Array(w263, w262) -> (w259:i32[])
          n92 = in-place {
            in-place-border: w258 -> [w267]
            in-place-border: LVMapReplaceAction."Modify Entry only if found" ("action") -> [w265]
            n93 = in-place-map #5(w261, w259) -> (w268:dbl)  [unwired: 1 in, 1 out]
            n94 = Divide(x=w268, y=w267) -> (x/y=w266:cdb)
            n95 = in-place-map #5(w266, w265) -> (w260:map{i32[], dbl})  [unwired: 2 out]
          }
        }
      }
      n96 = for {
        shift-right: [w304] -> w233
        shift-left: map{i32, dbl} {} ("parameters IN") -> [w305]
        tunnel: w216 -> [w303] mode=indexing
        shift-right: [w302] -> w217
        shift-left: w237 -> [w302]
        n97 = Unbundle(w303) -> ("index"=w300:i32, "X selector"=w301:T2)
        n98 = Look In Map(map=w302, key=w301) -> (value=w299:dbl)  [unwired: 1 in, 1 out]
        n99 = Insert Into Map(map in=w305, key=w300, value=w299) -> (map out=w304:map{i32, dbl})  [unwired: 2 out]
      }
      n100 = Collection Size(1:w216) -> (0:w224:i32)
      n101 = Initialize Array(0.0 ("number"), w224, w224) -> (w228:dbl[][])
      n102 = Initialize Array(0.0 ("number"), w224) -> (w231:dbl[])
      n103 = for {
        tunnel: w216 -> [w280] mode=indexing
        tunnel: w216 -> [w281]
        shift-right: [w278] -> w225
        shift-left: w235 -> [w279]
        shift-right: [w277] -> _
        shift-left: w233 -> [w275]
        shift-right: [w271] -> w229
        shift-left: w231 -> [w276]
        shift-right: [w270] -> w227
        shift-left: w228 -> [w269]
        n104 = Unbundle(w280) -> ("index"=w274:i32)  [unwired: 1 out]
        n105 = Look In Map(map=w275, key=w274) -> (value=w272:dbl)  [unwired: 1 in, 1 out]
        n106 = Decrement(x=w274) -> (x-1=w273:i32)
        n107 = Replace Array Subset(array=w276, new element=w272, index=w273) -> (w271:dbl[])
        n108 = for {
          tunnel: w281 -> [w298] mode=indexing
          tunnel: w274 -> [w287]
          shift-right: [w290] -> w278
          shift-left: w279 -> [w291]
          shift-right: [w297] -> w277
          shift-left: w275 -> [w297]
          shift-right: [w288] -> w270
          shift-left: w269 -> [w282]
          n109 = Unbundle(w298) -> ("index"=w286:i32)  [unwired: 1 out]
          n110 = Build Array(w287, w286) -> (w289:i32[])
          n111 = Look In Map(map=w297, key=w286) -> (value=w295:dbl)  [unwired: 1 in, 1 out]
          n112 = Look In Map(map=w297, key=w287) -> (value=w296:dbl)  [unwired: 1 in, 1 out]
          n113 = Look In Map(map=w291, key=w289) -> (value=w293:dbl)  [unwired: 1 in, 1 out]
          n114 = Compound Arithmetic op=MULTIPLY(-1.0 ("value"), w295, w296) -> (w292:dbl)
          n115 = Decrement(x=w286) -> (x-1=w285:i32)
          n116 = Decrement(x=w287) -> (x-1=w284:i32)
          n117 = Compound Arithmetic op=ADD(w293, w292) -> (w283:dbl)
          n118 = Replace Array Subset(array=w282, new element=w283, index (row)=w285, index (col)=w284) -> (w288:dbl[][])
          n119 = Insert Into Map(map in=w291, key=w289, value=w283) -> (map out=w290:map{i32[], dbl})  [unwired: 2 out]
        }
      }
      "d2G / d log α d log  β  map  OUT" <- w225
      n120 = call-poly <vilib>:"Array To Matrix.vi"("Real 1D Array"=w229) -> ("Real Matrix (Column Vector)"=w208:T7)
      n121 = call-poly <vilib>:"Array To Matrix.vi"("Real 2D Array"=w227) -> ("Real Matrix"=w211:T7)
      n122 = call-poly <vilib>:"Inverse Matrix.vi"("matrix type"=Matrix_Type_of_Inverse_Matrix."General", "Input Matrix"=w211) -> ("Inverse Matrix"=w210:T7)  [unwired: 1 out]
      n123 = call-poly <vilib>:"A x B.vi"("B"=w208, "A"=w210) -> ("A x B"=w209:T7)  [unwired: 1 out]
      n124 = call-poly <vilib>:"Matrix To Array.vi"("Real Matrix"=w209) -> ("Real 2D Array"=w221:dbl[][])
      n125 = call-poly <vilib>:"Matrix Norm.vi"("norm type"=w223, "Input Matrix"=w209) -> ("norm"=w220:dbl)  [unwired: 1 out]
      n126 = call-poly <vilib>:"Matrix Norm.vi"("norm type"=w222, "Input Matrix"=w208) -> ("norm"=w218:dbl)  [unwired: 1 out]
      n127 = Divide(x=w221, y=w220) -> (x/y=w219:dbl[][])
      n128 = Multiply(x=w219, y=w218) -> (x*y=w214:dbl[][])
      n129 = Multiply(x=w214, y=-1.0) -> (x*y=w212:dbl[][])
      n130 = for {
        tunnel: w216 -> [w242] mode=indexing
        shift-right: [w243] -> w215
        shift-left: w217 -> [w244]
        tunnel: w212 -> [w240]
        n131 = Unbundle(w242) -> ("index"=w239:i32, "X selector"=w241:T2)
        n132 = in-place {
          in-place-border: w240 -> [w249]
          in-place-border: w239 -> [w248]
          n133 = in-place-map #6(w244, w241) -> ()  [unwired: 1 in, 2 out]
          n134 = Decrement(x=w248) -> (x-1=w247:i32)
          n135 = Index Array(array=w249, index (row)=w247, index (col)=0 ("disabled index (col)")) -> (element=w246:dbl)
          n136 = in-place-map #6(w246, LVMapReplaceAction."Modify Entry only if found" ("action")) -> (w243:map{T2, dbl})  [unwired: 2 out]
        }
      }
    }
  }
  "dG / d log α   OUT" <- w6
